vi "_JKISMQFGV.vi"(6 "?":T2, 8 "Error in":errorcluster caption="Error in (no error)", 9 "create if not found? (T)":bool=TRUE, 11 "Name(\"\" to use uuid) in":string) -> (0 "Error out":errorcluster, 1 "Boolean":bool, 2 "Name":string[](array[string]), 3 "Array":T1[](array[typedef]))   [LabVIEW 2014, in "JKI-State-Machine-Plus.lvlib"]
uses:
  JKI-State-Machine-Plus.lvlib
  _JKISMQFGVOPER.ctl
  _JKISMQ.ctl
  _Cross JKI StateMachine State Data.ctl
  _Cross JKI StateMachine State Response.ctl
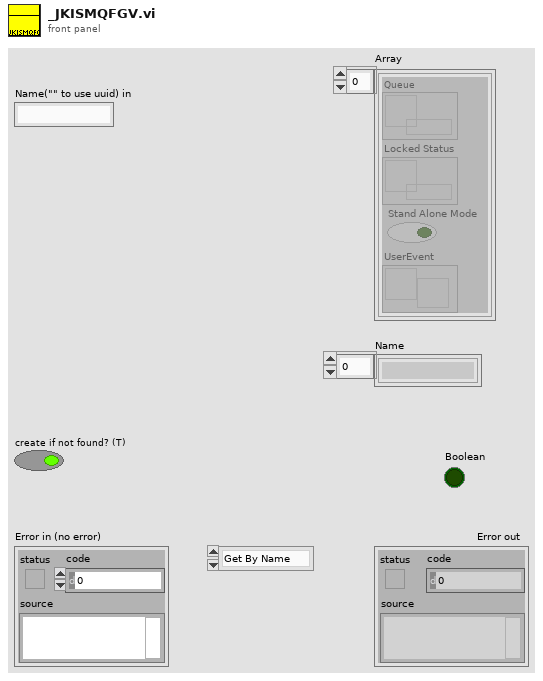
[diagram p1: front panel]
types:
  T1 = typedef "JKI-State-Machine-Plus.lvlib/_JKISMQ.ctl" = cluster{"Queue":refnum<queue>, "Locked Status":refnum<data-value>, "Stand Alone Mode":bool, "UserEvent":refnum<user-event>}
  T2 = typedef "JKI-State-Machine-Plus.lvlib/_JKISMQFGVOPER.ctl" = enum16{"Get By Name", "List", "Check If Name Exists"}
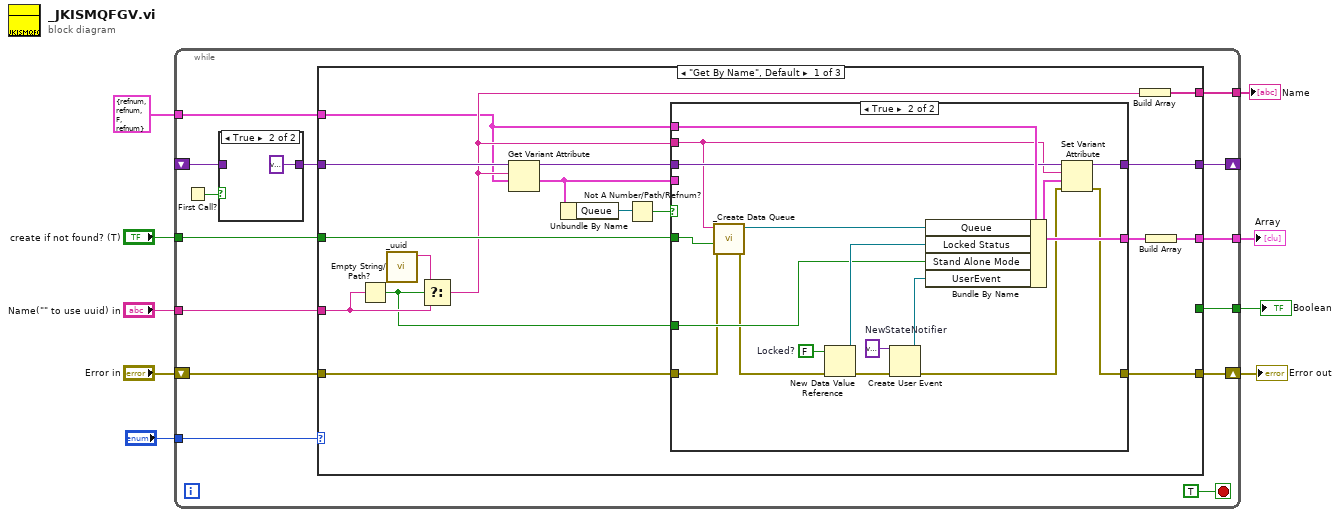
[diagram p0: block diagram]
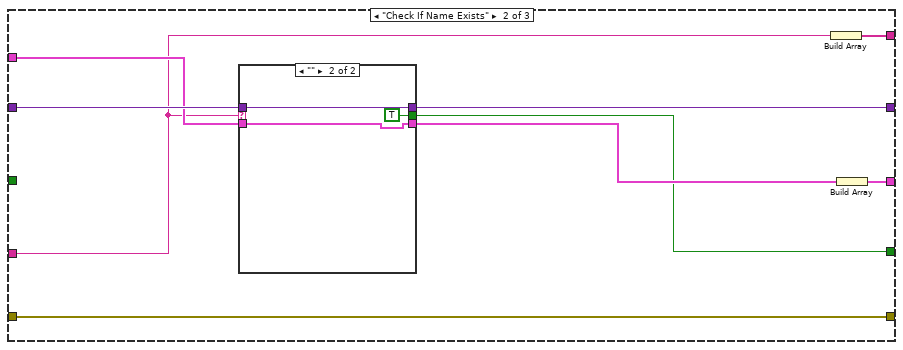
[diagram p4: hidden frame]
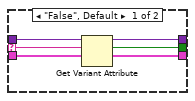
[diagram p5: hidden frame]
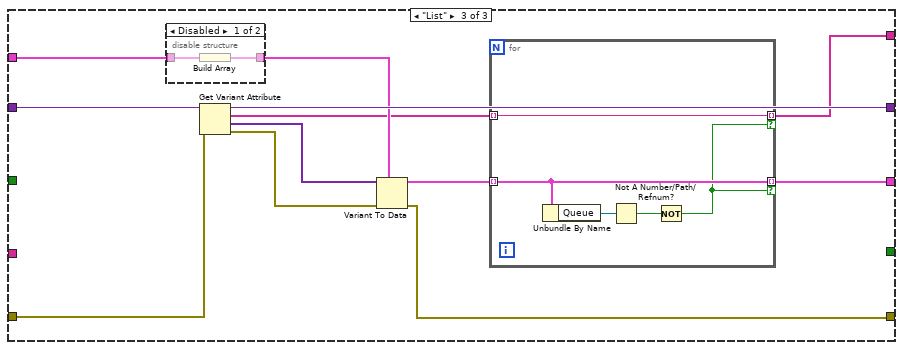
[diagram p6: hidden frame]
diagram:
  n1 = while {
    tunnel: "?" -> [w22]
    tunnel: "Name(\"\" to use uuid) in" -> [w21]
    tunnel: "create if not found? (T)" -> [w20]
    tunnel: [w19] -> w2
    shift-right: [w15] -> _
    shift-left: _ -> [w17]
    shift-right: [w13] -> w5
    shift-left: "Error in" -> [w14]
    tunnel: [w12] -> w4
    tunnel: T1 {"Queue"=refnum, "Locked Status"=refnum, "Stand Alone Mode"=FALSE, "UserEvent"=refnum} ("JKISMQ") -> [w11]
    tunnel: [w10] -> w1
    stop <- TRUE stop-if-true
    n2 = First Call?() -> (First Call?: T/F=w18:bool)
    n3 = case shown="True" w18 {
      tunnel: [w24 variant] -> w16
      tunnel: w17 -> [w24 _]
      frame False {
      }
      frame True {
      }
    }
    n4 = case shown="\"Get By Name\", Default" w22 {
      tunnel: w21 -> [w41 w64 _]
      tunnel: w20 -> [w40 _ _]
      tunnel: [w27 w66 w84] -> w19
      tunnel: w16 -> [w37 w71 w92]
      tunnel: [w35 w70 w91] -> w15
      tunnel: w14 -> [w31 w68 w82]
      tunnel: [w30 w68 w81] -> w13
      tunnel: [w26 w65 w85] -> w12
      tunnel: w11 -> [w28 w67 w89]
      tunnel: [_ w63 _] -> w10
      frame "Get By Name", Default {
        n5 = Empty String/Path?(string/path=w41) -> (empty?=w39:bool)
        n6 = call "_uuid.vi"() -> ("UUID"=w42:string)  [unwired: 11 in]
        n7 = Select(t=w42, s=w39, f=w41) -> (s? t:f=w29:string)
        n8 = Get Variant Attribute(Variant=w37, name=w29, default value (empty Variant)=w28) -> (duplicate Variant=w36:variant, value=w34:T1)  [unwired: 1 in, 2 out]
        n9 = Unbundle By Name(w34) -> ("Queue"=w33:refnum<queue>)
        n10 = Not A Number/Path/Refnum?(number/path/refnum=w33) -> (NaN/Path/Refnum?=w32:bool)
        n11 = case shown="True" w32 {
          tunnel: w40 -> [_ w61]
          tunnel: w39 -> [_ w58]
          tunnel: [w44 w53] -> w38
          tunnel: w29 -> [_ w54]
          tunnel: w28 -> [_ w57]
          tunnel: w36 -> [w45 w56]
          tunnel: [w45 w55] -> w35
          tunnel: w34 -> [w44 _]
          tunnel: w31 -> [w43 w52]
          tunnel: [w43 w50] -> w30
          frame False {
          }
          frame True {
            w49 = variant  # NewStateNotifier
            w62 = FALSE  # Locked?
            n12 = call "_Create Data Queue.vi"("error in (no error)"=w52, "create if not found? (T)"=w61, "Name"=w54) -> ("error out"=w51:errorcluster, "Queue out"=w60:refnum<queue>)  [unwired: 6 in, 1 out]
            n13 = New Data Value Reference(data value=w62, error in=w51) -> (data value reference=w59:refnum<data-value>, error out=w48:errorcluster)
            n14 = Create User Event(user event datatype=w49, error in=w48) -> (user event=w47:refnum<user-event>, error out=w46:errorcluster)
            n15 = Bundle By Name(cluster=w57, "Queue"=w60, "Locked Status"=w59, "Stand Alone Mode"=w58, "UserEvent"=w47) -> (w53:T1)
            n16 = Set Variant Attribute(Variant=w56, name=w54, value=w53, error in=w46) -> (Variant out=w55:variant, error out=w50:errorcluster)  [unwired: 1 out]
          }
        }
        n17 = Build Array(w29) -> (w26:string[])
        n18 = Build Array(w38) -> (w27:T1[])
      }
      frame "Check If Name Exists" {
        n19 = case shown="\"\"" w64 {
          selector: w64 -> [w73 _]
          tunnel: w71 -> [w77 w80]
          tunnel: [w76 w80] -> w70
          tunnel: [w75 w78] -> w69
          tunnel: w67 -> [w74 w78]
          tunnel: [w72 TRUE] -> w63
          frame "False", Default {
            n20 = Get Variant Attribute(Variant=w77, name=w73, default value (empty Variant)=w74) -> (duplicate Variant=w76:variant, found=w72:bool, value=w75:T1)  [unwired: 1 in, 1 out]
          }
          frame "" {
          }
        }
        n21 = Build Array(w64) -> (w65:string[])
        n22 = Build Array(w69) -> (w66:T1[])
      }
      frame "List" {
        n23 = disable-structure shown="Disabled" {
          disable-tunnel: w89 -> [w99 _]
          disable-tunnel: [w98 _] -> w88
          frame Disabled {
            n24 = Build Array(w99) -> (w98:T1[])
          }
          frame Enabled {
          }
        }
        n25 = Get Variant Attribute(Variant=w92, error in=w82) -> (duplicate Variant=w91:variant, names=w86:string[], values=w90:variant[], error out=w83:errorcluster)  [unwired: 2 in]
        n26 = Variant To Data(error in=w83, type=w88, Variant=w90) -> (data=w87:T1[], error out=w81:errorcluster)
        n27 = for {
          tunnel: w87 -> [w96] mode=indexing
          tunnel: w86 -> [w97] mode=indexing
          tunnel: [w97] -> w85 mode=indexing if=w93
          tunnel: [w96] -> w84 mode=indexing if=w93
          n28 = Unbundle By Name(w96) -> ("Queue"=w95:refnum<queue>)
          n29 = Not A Number/Path/Refnum?(number/path/refnum=w95) -> (NaN/Path/Refnum?=w94:bool)
          n30 = Not(x=w94) -> (.not. x?=w93:bool)
        }
      }
    }
  }
  "Error out" <- w5
  "Name" <- w4
  "Array" <- w2
  "Boolean" <- w1
